vi "Configuration DVR Global.vi"() -> ()   [LabVIEW 2020, in "Performance Monitor UI.lvlib" / "Configuration.lvlib"]
doc: "Global access to the configuration DVR.\n_____\nBased on DCFG Project Template 1.0.0.21.\n____\nPeloton Config 1.0.0.2\nCopyright (c) 2022, Peloton"
uses:
  Configuration.lvlib
  Configuration--cluster.ctl
panel:
  out "Configuration DVR":refnum<data-value>
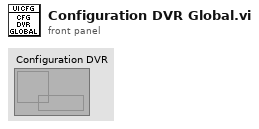
[diagram p1: front panel]
diagram:
